vi "Ramp Control.vi"(8 "Forward/Reverse":bool, 10 "Enum":T1) -> ()   [LabVIEW 2014]
uses:
  TypeDefs/SRE Enum.ctl
  <vilib>/Rock Robotics/WPI/Solenoid/WPI_SolenoidChannel.ctl
  <vilib>/Rock Robotics/WPI/Solenoid/WPI_SolenoidValue.ctl
  <vilib>/Rock Robotics/WPI/Solenoid/WPI_SolenoidOpenDouble.vi
  <vilib>/Rock Robotics/WPI/Solenoid/WPI_SolenoidSetEnum.vi
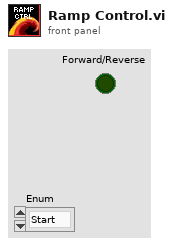
[diagram p1: front panel]
types:
  T1 = typedef "SRE Enum.ctl" = enum16{"Start", "Run", "End"}
  T2 = typedef "WPI_SolenoidChannel.ctl" = enum8{"Solenoid 0", "Solenoid 1", "Solenoid 2", "Solenoid 3", "Solenoid 4", "Solenoid 5", "Solenoid 6", "Solenoid 7", "Invalid"}
  T3 = typedef "WPI_SolenoidValue.ctl" = enum16{"Off", "On", "Forward", "Reverse"}
  T4 = typedef "WPI_SolenoidDevRef.ctl" = cluster{"DevStatus":errorcluster, "Pneumatics Control Module":u8, "Forward Solenoid Channel":T2, "Reverse Solenoid Channel":T2}
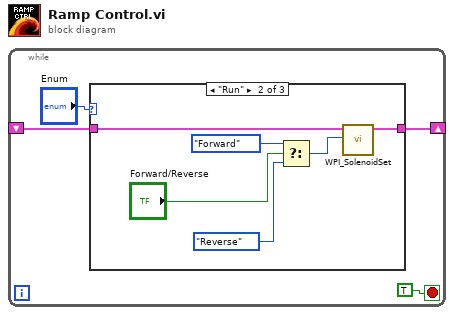
[diagram p0: block diagram]
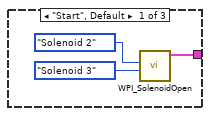
[diagram p2: hidden frame]
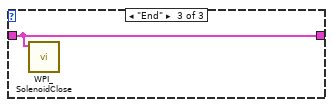
[diagram p3: hidden frame]
diagram:
  n1 = while {
    shift-right: [w3] -> _
    shift-left: _ -> [w2]
    stop <- TRUE stop-if-true
    n2 = case shown="\"Run\"" "Enum" {
      tunnel: [w7 w13 w14] -> w3
      tunnel: w2 -> [_ w12 w14]
      frame "Start", Default {
        n3 = call-poly <vilib>:"WPI_SolenoidOpen.vi"("Reverse Solenoid Channel"=WPI_SolenoidChannel."Solenoid 3", "Forward Solenoid Channel"=WPI_SolenoidChannel."Solenoid 2") -> ("SolenoidDevRef"=w7:T4)  [unwired: 8 in, 1 out]
      }
      frame "Run" {
        n4 = Select(t=WPI_SolenoidValue."Forward" ("Value"), s="Forward/Reverse", f=WPI_SolenoidValue."Reverse") -> (s? t:f=w10:T3)
        n5 = call-poly <vilib>:"WPI_SolenoidSet.vi"("Value"=w10, "SolenoidDevRef"=w12) -> ("SolenoidDevRef"=w13:T4)  [unwired: 8 in, 1 out]
      }
      frame "End" {
        n6 = call <vilib>:"WPI_SolenoidClose.vi"("SolenoidDevRef"=w14) -> ()  [unwired: 10 in, 1 out]
      }
    }
  }
